vi "circle_fit.vi"() -> ()   [LabVIEW 2024]
uses:
  <vilib>/Utility/file.llb/Read Delimited Spreadsheet (DBL).vi
  <vilib>/Analysis/1siggen.llb/Ramp Pattern by Samples.vi
  <vilib>/gmath/NI_Gmath.lvlib
  <vilib>/Analysis/NI_AALBase.lvlib
panel:
  out "column2":dbl[][](array[numeric])
  out "column1":dbl[][](array[numeric])
  out "all rows":dbl[][](array[numeric])
  in  "file (use dialog)":path
  out "center":cdb format="%.4f"
  out "r":dbl format="%.4f"
  out "XY Graph":cluster{cdb[]}[](graph)
  # "Read Magnetometer data from rotating the magnetometer 360 degrees in the horizontal plane"
  # "For Troubleshoot"
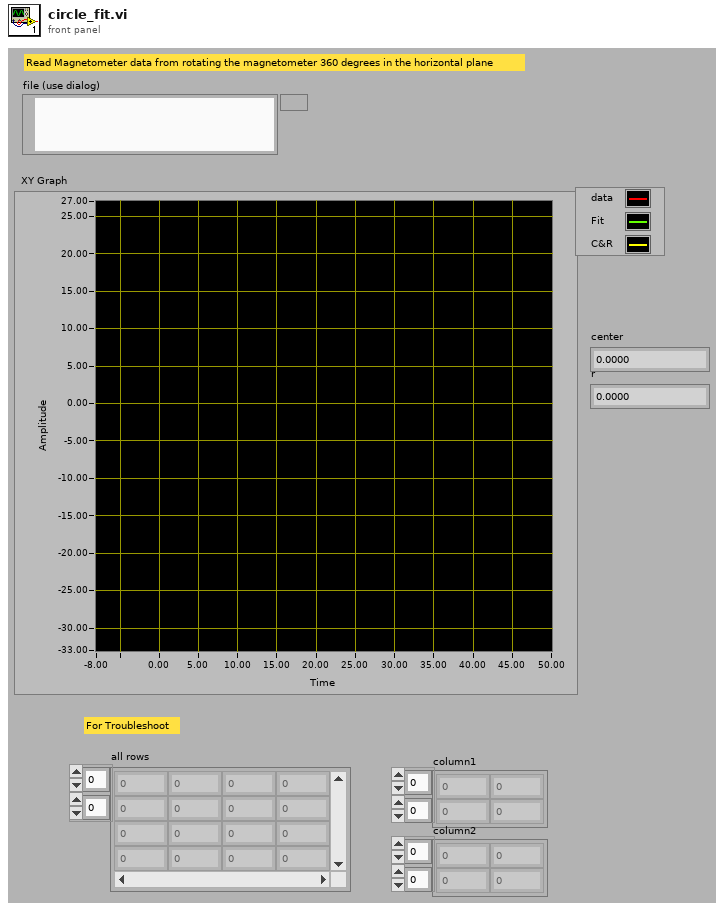
[diagram p1: front panel]
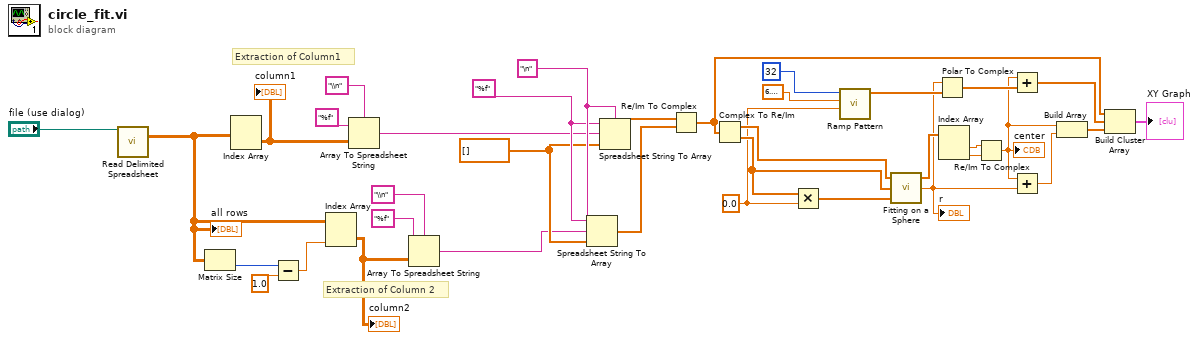
[diagram p0: block diagram]
diagram:
  w18 = 0.0 ("start")
  w36 = "\n" ("delimiter (Tab)")
  w35 = "%f" ("spreadsheet string")
  w33 = dbl[] [] ("array type (2D Dbl)")
  # "Extraction of Column 2"
  # "Extraction of Column1"
  n1 = call-poly <vilib>:"Read Delimited Spreadsheet.vi"("file path (dialog if empty)"="file (use dialog)") -> ("all rows"=w12:dbl[][])  [unwired: 9 in, 5 out]
  "all rows" <- w12
  n2 = Matrix Size(0:w12) -> (2:w9:i32)  [unwired: 1 out]
  n3 = Index Array(array=w12) -> (element=w8:dbl[][])  [unwired: 2 in]
  "column1" <- w8
  n4 = Subtract(x=w9, y=1.0) -> (x-y=w10:dbl)
  n5 = Index Array(array=w12, index (col)=w10) -> (element=w4:dbl[][])  [unwired: 1 in]
  "column2" <- w4
  n6 = Array To Spreadsheet String(delimiter (Tab)="\\n", array=w8, 3:"%f" ("format string")) -> (spreadsheet string=w2:string)
  n7 = Array To Spreadsheet String(delimiter (Tab)="\\n", array=w4, 3:"%f" ("format string")) -> (spreadsheet string=w1:string)
  n8 = Spreadsheet String To Array(delimiter (Tab)=w36, format string=w35, spreadsheet string=w1, array type (2D Dbl)=w33) -> (array=w28:dbl[])
  n9 = Spreadsheet String To Array(delimiter (Tab)=w36, format string=w35, spreadsheet string=w2, array type (2D Dbl)=w33) -> (array=w29:dbl[])
  n10 = Re/Im To Complex(1:w28, 2:w29) -> (0:w27:cdb[])
  n11 = Complex To Re/Im(x + iy=w27) -> (x=w26:dbl[], y=w24:dbl[])
  n12 = Multiply(x=w24, y=w18) -> (x*y=w25:dbl[])
  n13 = call-poly <vilib>:"Ramp Pattern.vi"("start"=w18, "end"=6.283185307179586, "samples"=32) -> ("Ramp Pattern"=w30:dbl[])  [unwired: 7 in, 1 out]
  n14 = call <vilib>:"Fitting on a Sphere.vi"("Z"=w25, "Y"=w24, "X"=w26) -> ("r"=w14:dbl, "x0, y0, z0"=w21:dbl[])  [unwired: 1 out]
  "r" <- w14
  n15 = Polar To Complex(1:w30, 2:w14) -> (0:w20:cdb[])
  n16 = Index Array(array=w21) -> (element #1=w22:dbl, element #2=w23:dbl)  [unwired: 2 in]
  n17 = Re/Im To Complex(1:w23, 2:w22) -> (0:w16:cdb)
  "center" <- w16
  n18 = Add(x=w16, y=w20) -> (x+y=w19:cdb[])
  n19 = Add(x=w16, y=w14) -> (x+y=w15:cdb)
  n20 = Build Array(w16, w15) -> (w17:cdb[])
  n21 = Build Cluster Array(w27, w19, w17) -> (→"XY Graph":cluster{cdb[]}[])
